vi "Set and Get Active Cell Size.vi"(6 "Active Cell In":T1 caption="活动单元格:活动单元格", 7 "Mode":T3, 8 "错误输入":errorcluster, 10 "CellSize In":T2 caption="CellSize", 11 "Mlistbox Ref":refnum<vi>) -> (0 "错误输出":errorcluster, 2 "CellSize Out":T2 caption="CellSize", 3 "Mlistbox Ref Dup":refnum<vi>)   [LabVIEW 2012, in "Mlistbox Tools.lvlib"]
uses:
  Mlistbox Tools.lvlib
  ListBox/Custom Type/Read and Write Mode.ctl
  <vilib>/Utility/miscctls.llb/LVBoundsTypeDef.ctl
  <vilib>/Utility/miscctls.llb/LVRowAndColumnTypeDef.ctl
  ListBox/Listbox Tool.lvlib
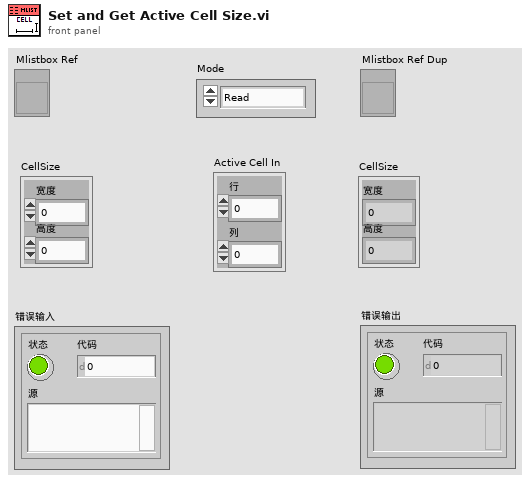
[diagram p1: front panel]
types:
  T1 = typedef "LVRowAndColumnTypeDef.ctl" = cluster{"Row":i32, "Column":i32}
  T2 = typedef "LVBoundsTypeDef.ctl" = cluster{"Width":u32, "Height":u32}
  T3 = typedef "Listbox Tool.lvlib/Read and Write Mode.ctl" = enum16{"Read", "Write"}
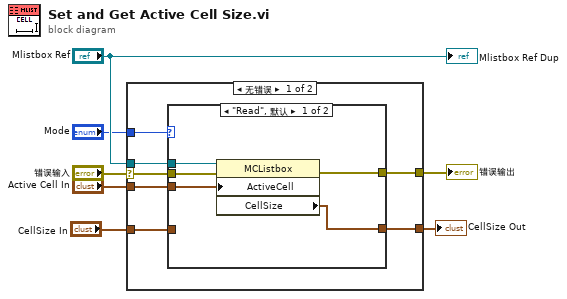
[diagram p0: block diagram]
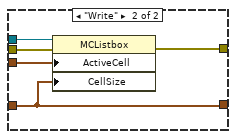
[diagram p2: hidden frame]
diagram:
  n1 = case shown="无错误" "错误输入" {
    selector: "错误输入" -> [w12 w25]
    tunnel: [w10 w25] -> w6
    tunnel: "Mlistbox Ref" -> [w13 _]
    tunnel: "Mode" -> [w14 _]
    tunnel: [w11 _] -> w3
    tunnel: "CellSize In" -> [w9 _]
    tunnel: "Active Cell In" -> [w8 _]
    frame No Error {
      n2 = case shown="\"Read\", 默认" w14 {
        tunnel: w13 -> [w19 w24]
        tunnel: w12 -> [w18 w23]
        tunnel: [w16 w21] -> w11
        tunnel: [w17 w22] -> w10
        tunnel: w9 -> [_ w21]
        tunnel: w8 -> [w15 w20]
        frame "Read", Default {
          n3 = property class="MCListbox"(reference=w19, error in=w18, "ActiveCell"=w15) -> (error out=w17:errorcluster, "CellSize"=w16:T2)  [unwired: 1 out]
        }
        frame "Write" {
          n4 = property class="MCListbox"(reference=w24, error in=w23, "ActiveCell"=w20, "CellSize"=w21) -> (error out=w22:errorcluster)  [unwired: 1 out]
        }
      }
    }
    frame Error {
    }
  }
  "错误输出" <- w6
  "CellSize Out" <- w3
  "Mlistbox Ref Dup" <- "Mlistbox Ref"
